vi "Create Enum Annotations.vi"(7 "error in (no error)":errorcluster, 10 "Enum Reference":refnum<vi>) -> (0 "error out":errorcluster, 2 "Annotations":string, 3 "Reference out":refnum<vi>)   [LabVIEW 2021, in "MeasurementLink Measurement Server.lvlib"]
uses:
  MeasurementLink Measurement Server.lvlib
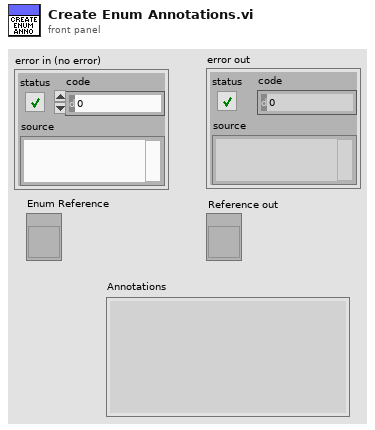
[diagram p1: front panel]
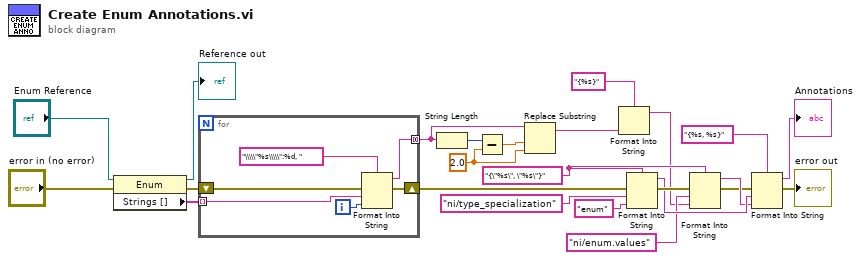
[diagram p0: block diagram]
diagram:
  w3 = 2.0 ("y")
  w19 = "{\"%s\", \"%s\"}" ("format string")
  n1 = property class="Enum"(reference="Enum Reference", error in="error in (no error)") -> (reference out=→"Reference out":refnum<vi>, error out=w9:errorcluster, "Strings []"=w11:string[])
  n2 = for {
    tunnel: w11 -> [w29] mode=indexing
    tunnel: [w27] -> w1 mode=concatenating
    shift-right: [w26] -> w13
    shift-left: w9 -> [w25]
    i -> [w28]
    n3 = Format Into String(format string="\\\\\"%s\\\\\":%d, ", error in=w25, w29, w28) -> (resulting string=w27:string, error out=w26:errorcluster)  [unwired: 1 in]
  }
  n4 = String Length(string=w1) -> (length=w5:i32)
  n5 = Subtract(x=w5, y=w3) -> (x-y=w4:dbl)
  n6 = Replace Substring(2:w3, 3:w4, 5:w1) -> (1:w2:string)  [unwired: 1 in, 1 out]
  n7 = Format Into String(format string="{%s}", w2) -> (resulting string=w6:string)  [unwired: 2 in, 1 out]
  n8 = Format Into String(format string=w19, error in=w13, "ni/type_specialization", "enum") -> (resulting string=w21:string, error out=w22:errorcluster)  [unwired: 1 in]
  n9 = Format Into String(format string=w19, error in=w22, "ni/enum.values", w6) -> (resulting string=w20:string, error out=w18:errorcluster)  [unwired: 1 in]
  n10 = Format Into String(format string="{%s, %s}", error in=w18, w21, w20) -> (resulting string=→"Annotations":string, error out=→"error out":errorcluster)  [unwired: 1 in]
